vi "智能门禁监测.vi"() -> ()   [LabVIEW 2016, in "环境动力监测库.lvlib" / "智能门禁监测.lvlib"]
uses:
  <vilib>/Utility/miscctls.llb/LVPointTypeDef.ctl
  <vilib>/Utility/config.llb/NI_LVConfig.lvlib
panel:
  out "SN":string
  out "write":string
  out "通信":bool
  out "read":string
  in  "输入簇":T1={"监测项描述:输出"="", "连接方式"=enum."串口", "端口"="", "IP address:"="", "Port:"="", "站号"=19200, "传感器型号"="", "波特率"=19200, "data bits"=8, "停止位"=10, "奇偶校验"=0, "声光告警启用"=FALSE} {"停止位" items=["1.0"=10, "1.5"=15, "2.0"=20]; "奇偶校验" items=["None", "Odd", "Even", "Mark", "Space"]}
  in  "卡号信息":i32[](listbox)=[0]
  in  "更新权限":bool
  out "门禁":bool
  in  "控制开关":bool caption="远程开门"
  # "智能门禁监测"
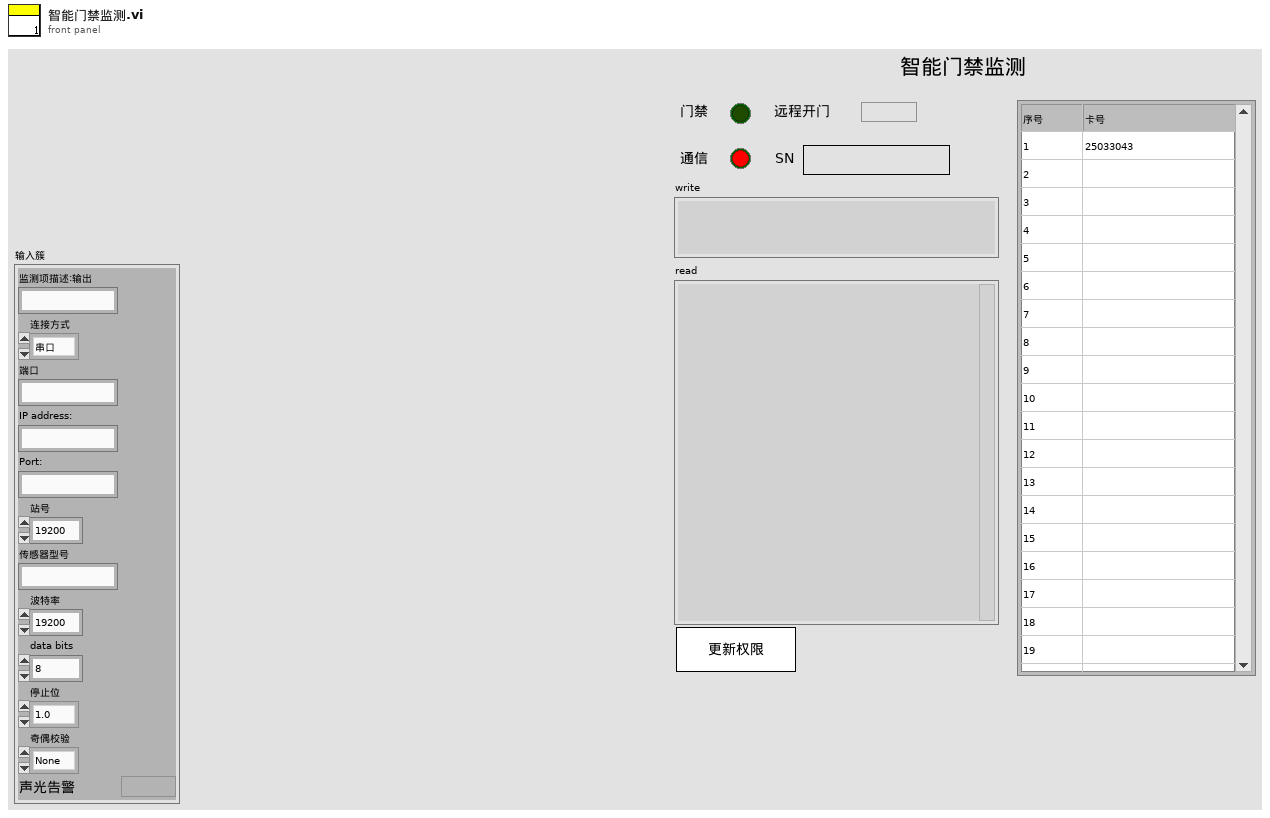
[diagram p1: front panel]
types:
  T1 = cluster{"监测项描述:输出":string, "连接方式":enum16{"串口", "TCP"}, "端口":string, "IP address:":string, "Port:":string, "站号":u64, "传感器型号":string, "波特率":u64, "data bits":u64, "停止位":u16, "奇偶校验":u16, "声光告警启用":bool}
  T2 = typedef "LVPointTypeDef.ctl" = cluster{"Horizontal":i16, "Vertical":i16}
  T3 = cluster{"choice":enum16{"open", "read", "write", "close"}, "write":string}
  T4 = typedef "NI_LVConfig.lvlib/Config Data RefNum.ctl" = refnum<k1>
  T5 = enum16{"Standard", "Buffered", "CRLF", "Immediate"}
  T6 = enum8{"Enabled", "Disabled", "Disabled and Grayed Out"}
  T7 = typedef "LVPoint32TypeDef.ctl" = cluster{"Horizontal":i32, "Vertical":i32}
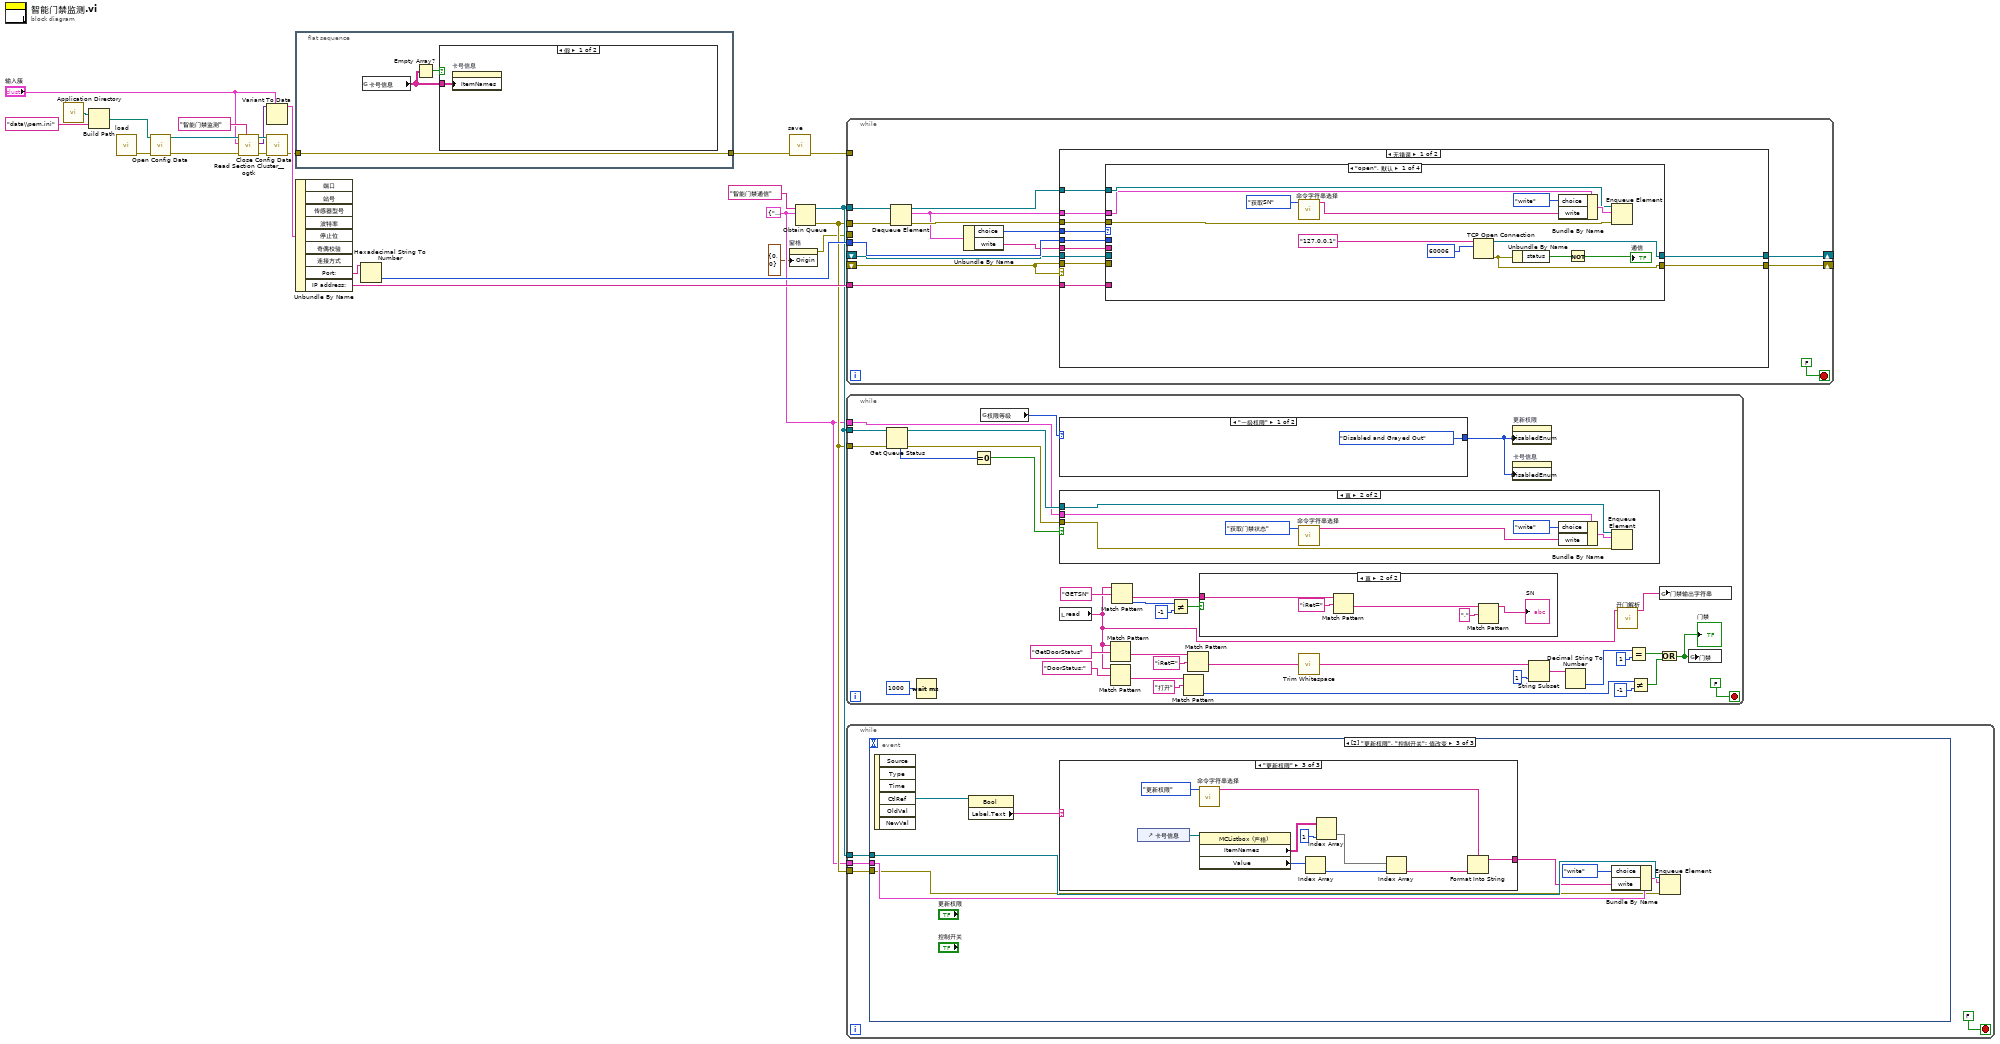
[diagram p0: block diagram]
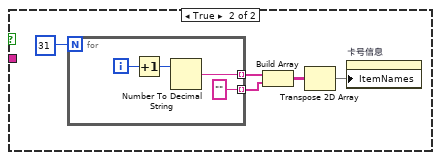
[diagram p2: hidden frame]
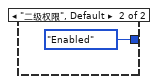
[diagram p4: hidden frame]
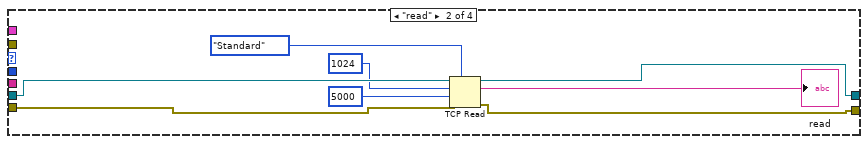
[diagram p6: hidden frame]
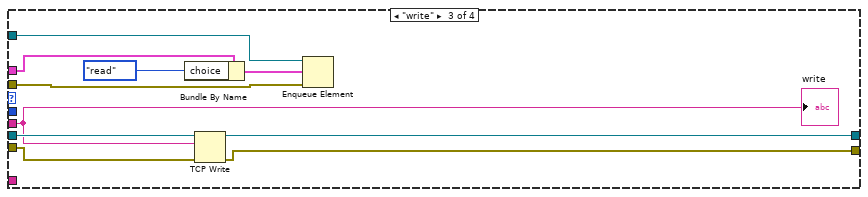
[diagram p7: hidden frame]
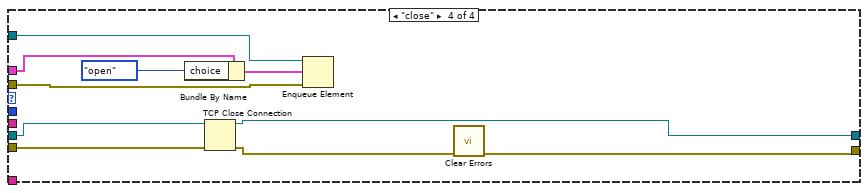
[diagram p8: hidden frame]
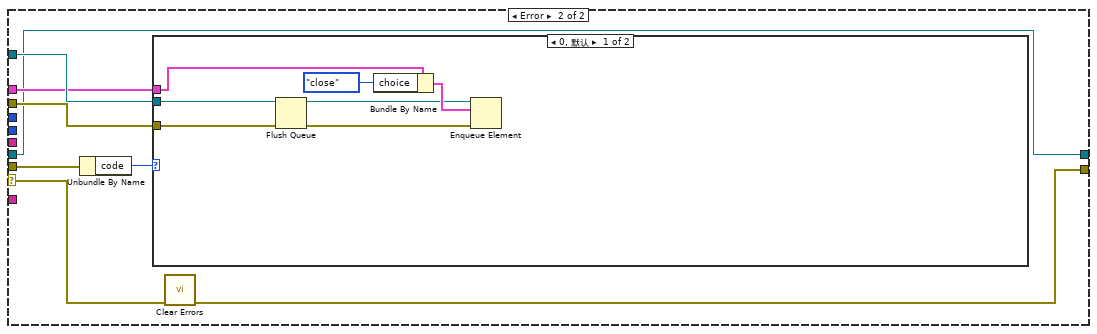
[diagram p9: hidden frame]
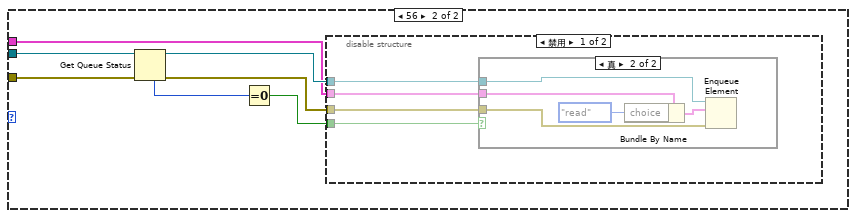
[diagram p10: hidden frame]
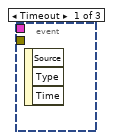
[diagram p13: hidden frame]
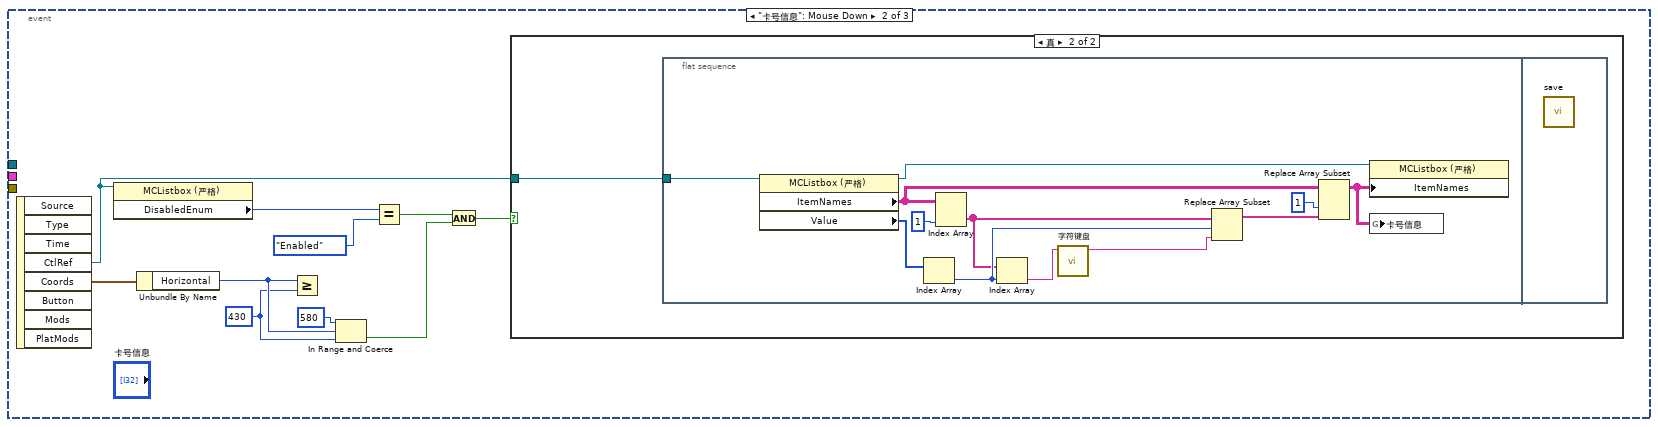
[diagram p14: hidden frame]
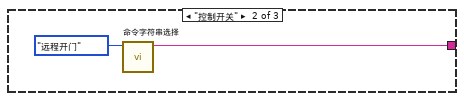
[diagram p17: hidden frame]
diagram:
  w5 = T3 {"choice"=enum."open", "write"=""}
  n1 = call <vilib>:"Application Directory.vi"() -> ("Application Directory"=w21:path)
  n2 = Build Path(base path=w21, name or relative path="data\\pem.ini" ("名称或相对路径")) -> (appended path=w22:path)
  n3 = call "load.vi"() -> ("error out"=w14:errorcluster)  [unwired: 11 in]
  n4 = call <vilib>:"Open Config Data.vi"("error in (no error)"=w14, "configuration file path"=w22) -> ("error out"=w23:errorcluster, "refnum"=w24:T4)  [unwired: 7 in, 1 out]
  n5 = call <userlib>:"Read Section Cluster__ogtk.vi"("section (optional)"="智能门禁监测", "error in (no error)"=w23, "Section Formatted Cluster Type"="输入簇", "refnum"=w24) -> ("error out"=w17:errorcluster, "Section Formatted Cluster"=w16:variant, "dup refnum"=w18:T4)  [unwired: 3 in, 2 out]
  n6 = Variant To Data(type="输入簇", Variant=w16) -> (data=w13:T1)  [unwired: 1 in, 1 out]
  n7 = call <vilib>:"Close Config Data.vi"("error in (no error)"=w17, "refnum"=w18) -> ("error out"=w4:errorcluster)  [unwired: 8 in, 1 out]
  n8 = flat-sequence {
    tunnel: w4 -> [w27]
    tunnel: [w27] -> w3
    frame #0 {
      n9 = global read "断电保存全局变量.vi" "卡号信息"() -> (w25:string[][])
      n10 = Empty Array?(array=w25) -> (empty?=w26:bool)
      n11 = case shown="假" w26 {
        tunnel: w25 -> [w28 _]
        frame False {
          n12 = property on="卡号信息" class="MCListbox (严格)"("ItemNames"=w28) -> ()  [unwired: 2 in, 2 out]
        }
        frame True {
          n13 = for {
            N: 31 -> [_]
            tunnel: [w36] -> w32 mode=indexing
            tunnel: [""] -> w29 mode=indexing
            i -> [w37]
            n14 = Increment(x=w37) -> (x+1=w35:i32)
            n15 = Number To Decimal String(number=w35) -> (decimal integer string=w36:string)  [unwired: 1 in]
          }
          n16 = Build Array(w32, w29) -> (w31:string[][])
          n17 = Transpose 2D Array(2D array=w31) -> (transposed array=w30:string[][])
          n18 = property on="卡号信息" class="MCListbox (严格)"("ItemNames"=w30) -> ()  [unwired: 2 in, 2 out]
        }
      }
    }
  }
  n19 = Unbundle By Name(w13) -> ("Port:"=w11:string, "IP address:"=w12:string)  [unwired: 7 out]
  n20 = Hexadecimal String To Number(string=w11) -> (number=w10:u32)  [unwired: 2 in, 1 out]
  n21 = property on="窗格" class="Pane"("Origin"=T2 {"Horizontal"=0, "Vertical"=0} ("原点")) -> (error out=w1:errorcluster)  [unwired: 2 in, 1 out]
  n22 = call "save.vi"("error in (no error)"=w3) -> ("error out"=w8:errorcluster)  [unwired: 10 in]
  n23 = Obtain Queue(name (unnamed)="智能门禁通信" ("名称（未命名）"), element data type=w5) -> (queue out=w7:refnum<queue>, error out=w6:errorcluster)  [unwired: 3 in, 1 out]
  n24 = while {
    tunnel: w8 -> [_]
    tunnel: w12 -> [w51]
    tunnel: w10 -> [w50]
    shift-right: [w49] -> _
    shift-left: _ -> [w48]
    shift-right: [w46] -> _
    shift-left: _ -> [w47]
    tunnel: w7 -> [w44]
    tunnel: w6 -> [w43]
    tunnel: w1 -> [_]
    stop <- FALSE stop-if-true
    n25 = Dequeue Element(queue=w44, error in (no error)=w43) -> (queue out=w40:refnum<queue>, element=w38:T3, error out=w39:errorcluster)  [unwired: 1 in, 1 out]
    n26 = Unbundle By Name(w38) -> ("choice"=w42:enum16{"open", "read", "write", "close"}, "write"=w41:string)
    n27 = case shown="无错误" w47 {
      selector: w47 -> [_ w106]
      tunnel: w42 -> [w62 _]
      tunnel: w51 -> [w61 _]
      tunnel: w50 -> [w60 _]
      tunnel: [w59 w104] -> w49
      tunnel: [w58 w105] -> w46
      tunnel: w48 -> [w57 w104]
      tunnel: w47 -> [w56 w111]
      tunnel: w41 -> [w55 _]
      tunnel: w40 -> [w54 w109]
      tunnel: w39 -> [w53 w108]
      tunnel: w38 -> [w52 w107]
      frame No Error {
        n28 = case shown="\"open\", 默认" w62 {
          tunnel: w61 -> [_ _ _ _]
          tunnel: w60 -> [_ _ _ _]
          tunnel: [w75 w81 w91 w101] -> w59
          tunnel: [w70 w80 w90 w94] -> w58
          tunnel: w57 -> [_ w83 w93 w103]
          tunnel: w56 -> [_ w82 w92 w102]
          tunnel: w55 -> [_ _ w89 _]
          tunnel: w54 -> [w65 _ w86 w98]
          tunnel: w53 -> [w64 _ w84 w96]
          tunnel: w52 -> [w63 _ w85 w97]
          frame "open", Default {
            n29 = call "命令字符串选择.vi"("枚举"=enum16{"获取SN", "获取门禁状态", "远程开门", "更新权限"}."获取SN") -> ("字符串"=w66:string)  [unwired: 10 in]
            n30 = TCP Open Connection(address="127.0.0.1" ("地址"), remote port or service name=u16 60006 ("远程端口或服务名称")) -> (connection ID=w75:refnum<k5>, error out=w70:errorcluster)  [unwired: 3 in]
            n31 = Unbundle By Name(w70) -> ("status"=w71:bool)
            n32 = Bundle By Name(cluster=w63, "choice"=enum16{"open", "read", "write", "close"}."write", "write"=w66) -> (w67:T3)
            n33 = Not(x=w71) -> (.not. x?=→"通信":bool)
            n34 = Enqueue Element(queue=w65, element=w67, error in (no error)=w64) -> ()  [unwired: 1 in, 3 out]
          }
          frame "read" {
            n35 = TCP Read(connection ID=w83, bytes to read=1024 ("读取的字节"), error in (no error)=w82, 7:T5."Standard" ("模式（标准）"), 9:5000 ("超时毫秒(25000)")) -> (connection ID out=w81:refnum<k5>, data out=→"read":string, error out=w80:errorcluster)
          }
          frame "write" {
            n36 = Bundle By Name(cluster=w85, "choice"=enum16{"open", "read", "write", "close"}."read") -> (w87:T3)
            n37 = TCP Write(connection ID=w93, data in=w89, error in (no error)=w92) -> (connection ID out=w91:refnum<k5>, error out=w90:errorcluster)  [unwired: 1 in, 1 out]
            n38 = Enqueue Element(queue=w86, element=w87, error in (no error)=w84) -> ()  [unwired: 1 in, 3 out]
            "write" <- w89
          }
          frame "close" {
            n39 = Bundle By Name(cluster=w97, "choice"=enum16{"open", "read", "write", "close"}."open") -> (w99:T3)
            n40 = TCP Close Connection(connection ID=w103, error in (no error)=w102) -> (connection ID out=w101:refnum<k5>, error out=w95:errorcluster)  [unwired: 1 in]
            n41 = Enqueue Element(queue=w98, element=w99, error in (no error)=w96) -> ()  [unwired: 1 in, 3 out]
            n42 = call <vilib>:"Clear Errors.vi"("error in (no error)"=w95) -> ("error out"=w94:errorcluster)  [unwired: 5 in, 1 out]
          }
        }
      }
      frame Error {
        n43 = Unbundle By Name(w111) -> ("code"=w110:i32)
        n44 = case shown="0, 默认" w110 {
          tunnel: w109 -> [w116 w122]
          tunnel: w108 -> [w113 w121]
          tunnel: w107 -> [w115 w120]
          frame 0, Default {
            n45 = Flush Queue(queue=w116, error in (no error)=w113) -> (queue out=w114:refnum<queue>, error out=w112:errorcluster)  [unwired: 1 out]
            n46 = Bundle By Name(cluster=w115, "choice"=enum16{"open", "read", "write", "close"}."close") -> (w117:T3)
            n47 = Enqueue Element(queue=w114, element=w117, error in (no error)=w112) -> ()  [unwired: 1 in, 3 out]
          }
          frame 56 {
            n48 = Get Queue Status(queue=w122, error in (no error)=w121) -> (queue out=w123:refnum<queue>, error out=w119:errorcluster, # elements in queue=w125:i32)  [unwired: 1 in, 5 out]
            n49 = Equal To 0?(x=w125) -> (x = 0?=w124:bool)
            n50 = disable-structure shown="禁用" {
              disable-tunnel: w124 -> [w129 _]
              disable-tunnel: w123 -> [w128 _]
              disable-tunnel: w120 -> [w127 _]
              disable-tunnel: w119 -> [w126 _]
              frame Disabled {
                n51 = case shown="真" w129 {
                  tunnel: w128 -> [_ w132]
                  tunnel: w127 -> [_ w131]
                  tunnel: w126 -> [_ w130]
                  frame False {
                  }
                  frame True {
                    n52 = Bundle By Name(cluster=w131, "choice"=enum16{"open", "read", "write", "close"}."read") -> (w133:T3)
                    n53 = Enqueue Element(queue=w132, element=w133, error in (no error)=w130) -> ()  [unwired: 1 in, 3 out]
                  }
                }
              }
              frame Enabled {
              }
            }
          }
        }
        n54 = call <vilib>:"Clear Errors.vi"("error in (no error)"=w106) -> ("error out"=w105:errorcluster)  [unwired: 5 in, 1 out]
      }
    }
  }
  n55 = while {
    tunnel: w7 -> [w167]
    tunnel: w6 -> [w166]
    tunnel: w5 -> [w161]
    stop <- FALSE stop-if-true
    n56 = Get Queue Status(queue=w167, error in (no error)=w166) -> (queue out=w163:refnum<queue>, error out=w162:errorcluster, # elements in queue=w165:i32)  [unwired: 1 in, 5 out]
    n57 = Wait (ms)(milliseconds to wait=u32 1000 ("等待时间（毫秒）")) -> ()  [unwired: 1 out]
    n58 = Equal To 0?(x=w165) -> (x = 0?=w164:bool)
    n59 = global read "外部交互全局变量.vi" "权限等级"() -> (w153:enum16{"一级权限", "二级权限", "三级权限", "超级权限"})
    n60 = case shown="\"一级权限\"" w153 {
      tunnel: [T6."Disabled and Grayed Out" ("禁用") T6."Enabled" ("禁用")] -> w152
      frame "一级权限" {
      }
      frame "二级权限", Default {
      }
    }
    n61 = case shown="真" w164 {
      tunnel: w163 -> [_ w183]
      tunnel: w162 -> [_ w182]
      tunnel: w161 -> [_ w181]
      frame False {
      }
      frame True {
        n62 = call "命令字符串选择.vi"("枚举"=enum16{"获取SN", "获取门禁状态", "远程开门", "更新权限"}."获取门禁状态") -> ("字符串"=w177:string)  [unwired: 10 in]
        n63 = Bundle By Name(cluster=w181, "choice"=enum16{"open", "read", "write", "close"}."write", "write"=w177) -> (w179:T3)
        n64 = Enqueue Element(queue=w183, element=w179, error in (no error)=w182) -> ()  [unwired: 1 in, 3 out]
      }
    }
    n65 = local read "read"() -> (w136:string)
    n66 = Match Pattern(string=w136, regular expression="GetDoorStatus") -> (after substring=w142:string)  [unwired: 1 in, 3 out]
    n67 = Match Pattern(string=w136, regular expression="DoorStatus:") -> (after substring=w150:string)  [unwired: 1 in, 3 out]
    n68 = Match Pattern(string=w136, regular expression="GETSN") -> (after substring=w141:string, offset past match=w138:i32)  [unwired: 1 in, 2 out]
    n69 = Not Equal?(x=w138, y=-1) -> (x != y?=w137:bool)
    n70 = Match Pattern(string=w150, regular expression="打开" ("正则表达式")) -> (offset past match=w148:i32)  [unwired: 1 in, 3 out]
    n71 = Match Pattern(string=w142, regular expression="iRet=" ("正则表达式")) -> (after substring=w159:string)  [unwired: 1 in, 3 out]
    n72 = case shown="真" w137 {
      tunnel: w141 -> [_ w174]
      frame False {
      }
      frame True {
        n73 = Match Pattern(string=w174, regular expression="iRet=" ("正则表达式")) -> (after substring=w172:string)  [unwired: 1 in, 3 out]
        n74 = Match Pattern(string=w172, regular expression="," ("正则表达式")) -> (before substring=→"SN":string)  [unwired: 1 in, 3 out]
      }
    }
    n75 = call <vilib>:"Trim Whitespace.vi"("string"=w159) -> ("trimmed string"=w158:string)  [unwired: 1 in]
    n76 = property on="更新权限" class="Bool (严格)"("DisabledEnum"=w152) -> ()  [unwired: 2 in, 2 out]
    n77 = property on="卡号信息" class="MCListbox (严格)"("DisabledEnum"=w152) -> ()  [unwired: 2 in, 2 out]
    n78 = String Subset(string=w158, length (rest)=1 ("长度（剩余）")) -> (substring=w156:string)  [unwired: 1 in]
    n79 = Decimal String To Number(string=w156) -> (number=w155:i32)  [unwired: 2 in, 1 out]
    n80 = call "开门解析.vi"("输入字符串"=w136) -> ("门禁输出字符串"=w135:string)  [unwired: 10 in]
    n81 = Equal?(x=w155, y=1) -> (x = y?=w146:bool)
    n82 = Not Equal?(x=w148, y=-1) -> (x != y?=w145:bool)
    n83 = Or(x=w146, y=w145) -> (x .or. y?=w144:bool)
    "门禁" <- w144
    n84 = global write "内部交互全局.vi" "门禁输出字符串"(w135) -> ()
    n85 = global write "内部交互全局.vi" "门禁"(w144) -> ()
  }
  n86 = while {
    tunnel: w7 -> [w186]
    tunnel: w6 -> [w185]
    tunnel: w5 -> [w184]
    stop <- FALSE stop-if-true
    n87 = event shown="[2] \"更新权限\", \"控制开关\": 值改变" {
      selector: _ -> [_ _ _]
      dyn-events: _ -> [_ _ _]
      timeout: _ -> [_ _ _]
      tunnel: w186 -> [_ _ w216]
      tunnel: w185 -> [_ _ w215]
      tunnel: w184 -> [_ _ w218]
      event Timeout {
        n88 = event-data() -> ()  [unwired: 1 in, 3 out]
      }
      event "卡号信息": Mouse Down {
        w195 = 430 ("y")
        n89 = event-data() -> ("CtlRef"=w191:refnum<vi>, "Coords"=w197:T7)  [unwired: 1 in, 6 out]
        n90 = property class="MCListbox (严格)"(reference=w191) -> ("DisabledEnum"=w190:T6)  [unwired: 1 in, 2 out]
        n91 = Unbundle By Name(w197) -> ("Horizontal"=w196:i32)
        n92 = Greater Or Equal?(x=w196, y=w195) -> ()  [unwired: 1 out]
        n93 = In Range and Coerce(upper limit=580 ("上限"), x=w196, lower limit=w195) -> (In Range?=w193:bool)  [unwired: 1 out]
        n94 = Equal?(x=w190, y=T6."Enabled") -> (x = y?=w188:bool)
        n95 = And(x=w188, y=w193) -> (x .and. y?=w192:bool)
        n96 = case shown="真" w192 {
          tunnel: w191 -> [_ w198]
          frame False {
          }
          frame True {
            n97 = flat-sequence {
              tunnel: w198 -> [w201]
              frame #0 {
                n98 = property class="MCListbox (严格)"(reference=w201) -> (reference out=w205:refnum<vi>, "ItemNames"=w206:string[][], "Value"=w210:i32[])  [unwired: 1 in, 1 out]
                n99 = Index Array(array=w210) -> (element=w204:i32)  [unwired: 1 in]
                n100 = Index Array(array=w206, index (col)=1 ("禁用的索引 (列)")) -> (element=w203:string[])  [unwired: 1 in]
                n101 = Index Array(array=w203, index=w204) -> (element=w200:string)
                n102 = call "字符键盘.vi"("原值"=w200) -> ("x+y"=w209:string)  [unwired: 10 in]
                n103 = Replace Array Subset(array=w203, new element=w209, index=w204) -> (w208:string[])
                n104 = Replace Array Subset(array=w206, new element=w208, index (col)=1 ("禁用的索引 (列)")) -> (w199:string[][])  [unwired: 1 in]
                n105 = property class="MCListbox (严格)"(reference=w205, "ItemNames"=w199) -> ()  [unwired: 1 in, 2 out]
                n106 = global write "断电保存全局变量.vi" "卡号信息"(w199) -> ()
              }
              frame #1 {
                n107 = call "save.vi"() -> ()  [unwired: 11 in, 1 out]
              }
            }
          }
        }
      }
      event "更新权限", "控制开关": Value Change {
        n108 = event-data() -> ("CtlRef"=w213:refnum<vi>)  [unwired: 1 in, 5 out]
        n109 = property class="Bool"(reference=w213) -> ("Label.Text"=w212:string)  [unwired: 1 in, 2 out]
        n110 = case shown="\"更新权限\"" w212 {
          tunnel: [_ w219 w223] -> w211
          frame "假", Default {
          }
          frame "控制开关" {
            n111 = call "命令字符串选择.vi"("枚举"=enum16{"获取SN", "获取门禁状态", "远程开门", "更新权限"}."远程开门") -> ("字符串"=w219:string)  [unwired: 10 in]
          }
          frame "更新权限" {
            n112 = control-ref of="卡号信息"() -> (w229:refnum<vi>)
            n113 = call "命令字符串选择.vi"("枚举"=enum16{"获取SN", "获取门禁状态", "远程开门", "更新权限"}."更新权限") -> ("字符串"=w221:string)  [unwired: 10 in]
            n114 = property class="MCListbox (严格)"(reference=w229) -> ("ItemNames"=w225:string[][], "Value"=w224:i32[])  [unwired: 1 in, 2 out]
            n115 = Index Array(array=w224) -> (element=w226:i32)  [unwired: 1 in]
            n116 = Index Array(array=w225, index (col)=1 ("禁用的索引 (列)")) -> (element=w227:string[])  [unwired: 1 in]
            n117 = Index Array(array=w227, index=w226) -> (element=w230:string)
            n118 = Format Into String(format string=w221, w230) -> (resulting string=w223:string)  [unwired: 2 in, 1 out]
          }
        }
        n119 = Bundle By Name(cluster=w218, "choice"=enum16{"open", "read", "write", "close"}."write", "write"=w211) -> (w214:T3)
        n120 = Enqueue Element(queue=w216, element=w214, error in (no error)=w215) -> ()  [unwired: 1 in, 3 out]
      }
    }
  }
